vi "Enable Display.vi"(8 "error in (no error)":errorcluster, 10 "Enable Display (T: Enable)":bool=TRUE, 11 "VISA resource name":refnum<visa-resource-name>) -> (0 "error out":errorcluster, 3 "VISA resource name out":refnum<visa-resource-name>)   [LabVIEW 2022 SP3, in "Keithley 24XX.lvlib"]
doc: "Enables or disables the display on the front of the instrument. Disabling the display can result in faster measurements."
uses:
  Keithley 24XX.lvlib
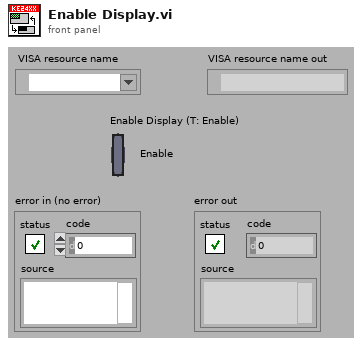
[diagram p1: front panel]
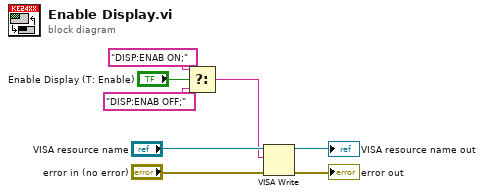
[diagram p0: block diagram]
diagram:
  n1 = Select(t="DISP:ENAB ON;", s="Enable Display (T: Enable)", f="DISP:ENAB OFF;") -> (s? t:f=w1:string)
  n2 = VISA Write(VISA resource name="VISA resource name", write buffer=w1, error in (no error)="error in (no error)") -> (VISA resource name out=→"VISA resource name out":refnum<visa-resource-name>, error out=→"error out":errorcluster)  [unwired: 1 out]
